vi "quiz3.vi"() -> ()   [LabVIEW 2020]
uses:
  <vilib>/Platform/TimedLoop/XDataNode/timing_clust.ctl
  <vilib>/Platform/TimedLoop/XDataNode/nitl_modes.ctl
  <vilib>/Platform/TimedLoop/XDataNode/wakeup.ctl
  enum.ctl
  <vilib>/Utility/file.llb/Read Delimited Spreadsheet (string).vi
  <vilib>/platform/TimedLoop/XDataNode/XDataNode.xnode
  <vilib>/Platform/TimedLoop/XDataNode/XDNodeRunTimeDep.lvlib
panel:
  out "Tab Control 2":enum32{"Login", "Registro", "Inicio"}(tab)
  in  "Enviar 2":bool
  in  "Usuario 2":string
  in  "Contraseña3":string
  out "Usuarios Eliminados 2":string[](array[string])
  out "Boolean 2":bool
  in  "Borrar Usuario 2":string
  in  "Usuario Nuevo 2":string
  in  "Clave de Usuario Nuevo 2":string
  in  "guardar 2":bool
  in  "Volver 2":bool
  in  "Borrar 2":bool
  in  "Volver a login 2":bool
  in  "Seleccione la secuencia":bool[][](array[boolean])
  out "Indicador por filas":bool[](array[boolean])
  out "Tab Control":enum32{"Login", "Registro", "Inicio"}(tab)
  in  "OK Button":bool
  in  "Usuario":string
  in  "Contraseña 2":string
  out "Boolean":bool
  in  "Borrar Usuario":string
  in  "Usuario Nuevo":string
  in  "Clave de Usuario Nuevo":string
  in  "guardar":bool
  in  "Volver":bool
  in  "Borrar":bool
  in  "Usuarios Eliminados":string[](array[string])
  in  "Volver a login":bool
  in  "Seleccione la secuencia":bool[][](array[boolean])
  out "Indicador por filas":bool[](array[boolean])
  # "Usuario"
  # "Contraseña"
  # "Usuarios Eliminados"
  # "Barrra de led interactiva"
  # "Contraseña"
  # "Barrra de led interactiva"
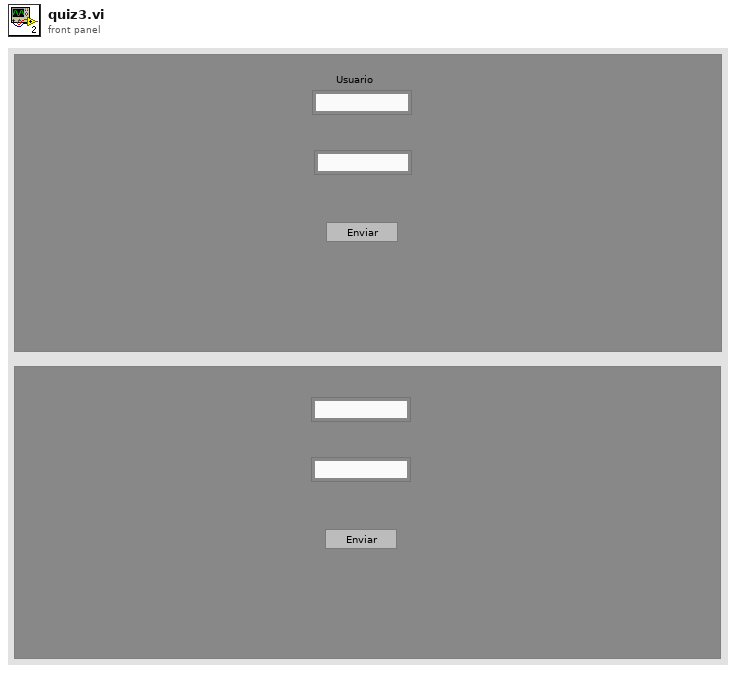
[diagram p1: front panel]
types:
  T1 = typedef "enum.ctl" = enum16{"login", "registro", "inicio"}
  T2 = enum16{"open", "replace", "create", "open or create", "replace or create", "replace or create with confirmation"}
  T3 = typedef "XDNodeRunTimeDep.lvlib/timing_clust.ctl" = cluster{"Expected End [f-1]":u64, "Actual End [f-1]":u64, "Finished Late? [f-1]":bool, "Expected End [i-1]":u64, "Actual End [i-1]":u64, "Finished Late? [i-1]":bool, "Expected Start [i]":u64, "Actual Start [i]":u64, "Expected Start [f]":u64, "Actual Start [f]":u64, "Source Name":string, "Structure Name":string, "Period":i64, "Deadline":i64, "Offset":i64, "Start":i64, "Priority":i32, "Timeout":i32, "Mode":T4, "Wakeup Reason":T5, "Error":errorcluster, "Source Type":string, "Secondary Source Type":string, "Global End Time":u64, "Global Start Time":u64, "Frame Duration":u64, "Iteration Duration":u64, "Assigned CPU":i32, "I/O Scan Engine Mode":u32}
  T4 = typedef "XDNodeRunTimeDep.lvlib/nitl_modes.ctl" = enum32{"No Change", "Process missed periods, maintain original phase", "Discard missed periods, maintain original phase", "Process missed periods, ignore original phase", "Discard missed periods, ignore original phase"}
  T5 = typedef "XDNodeRunTimeDep.lvlib/wakeup.ctl" = enum32{"Normal", "Aborted", "Asynchronous wakeup", "Timing source error", "Timed loop error", "Timeout"}
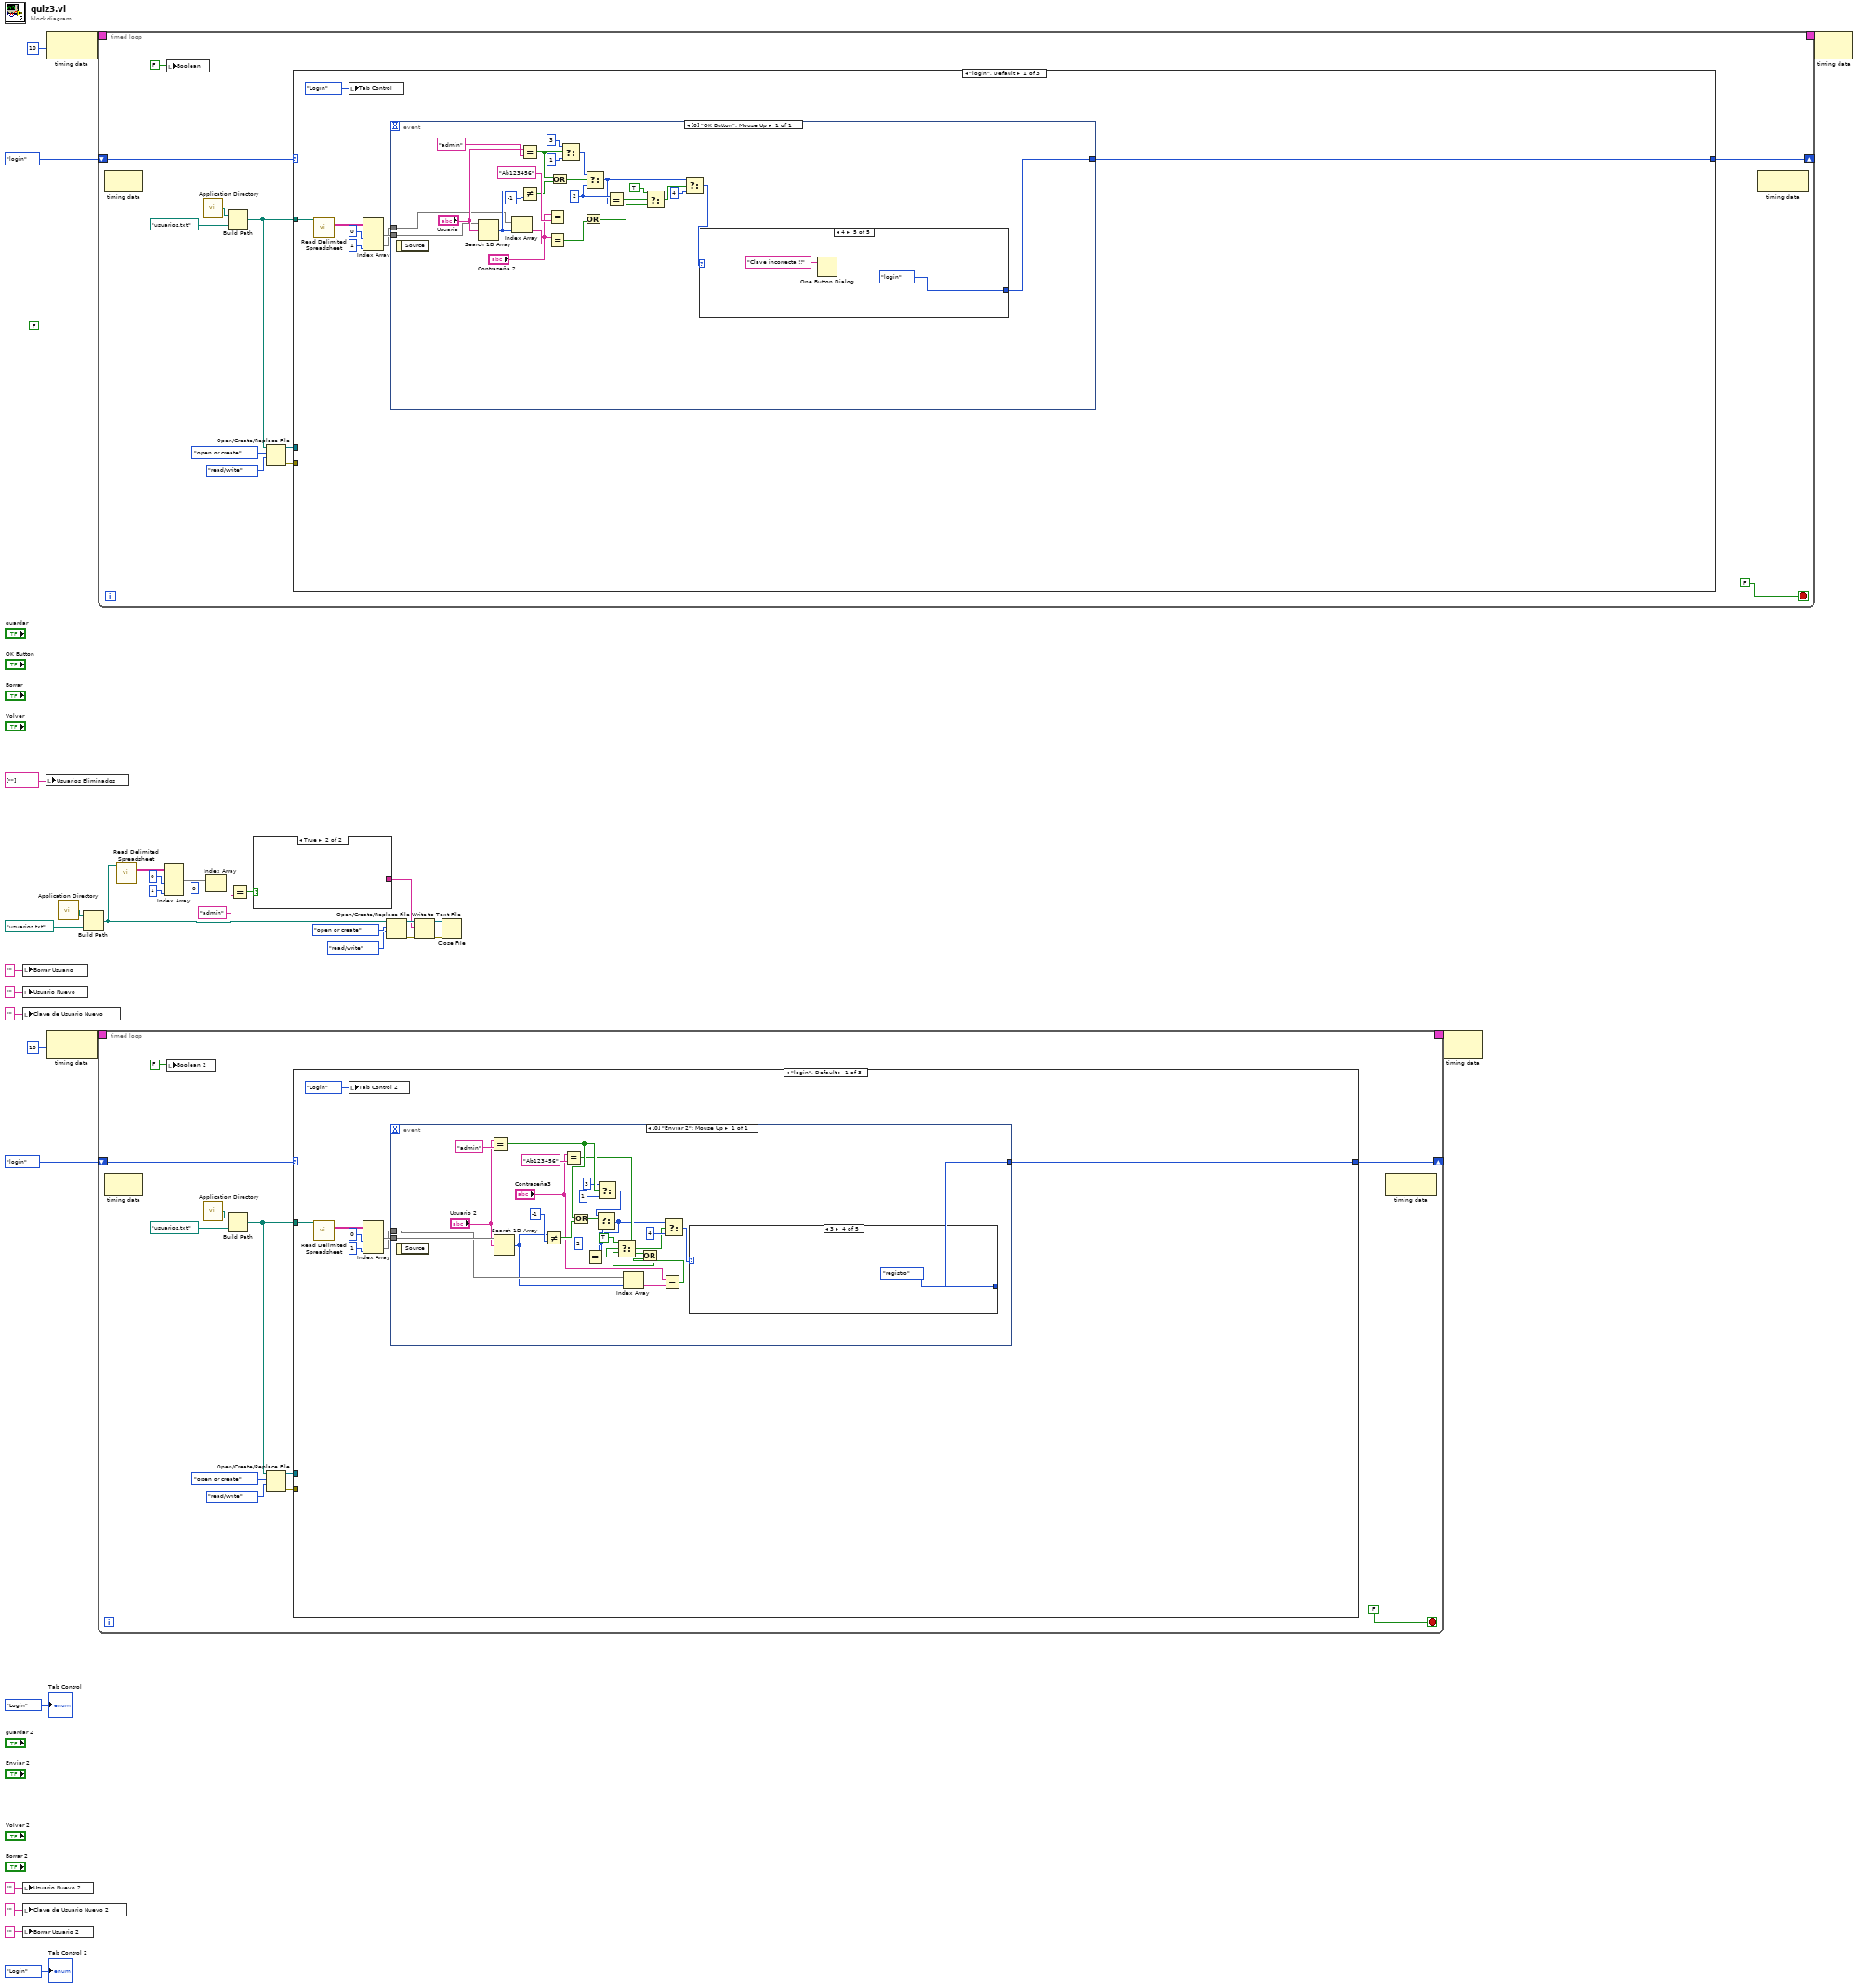
[diagram p0: block diagram]
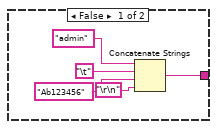
[diagram p2: hidden frame]
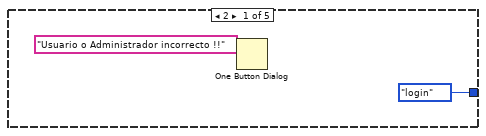
[diagram p3: hidden frame]
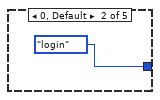
[diagram p4: hidden frame]
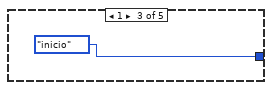
[diagram p5: hidden frame]
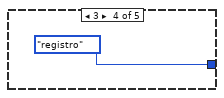
[diagram p6: hidden frame]
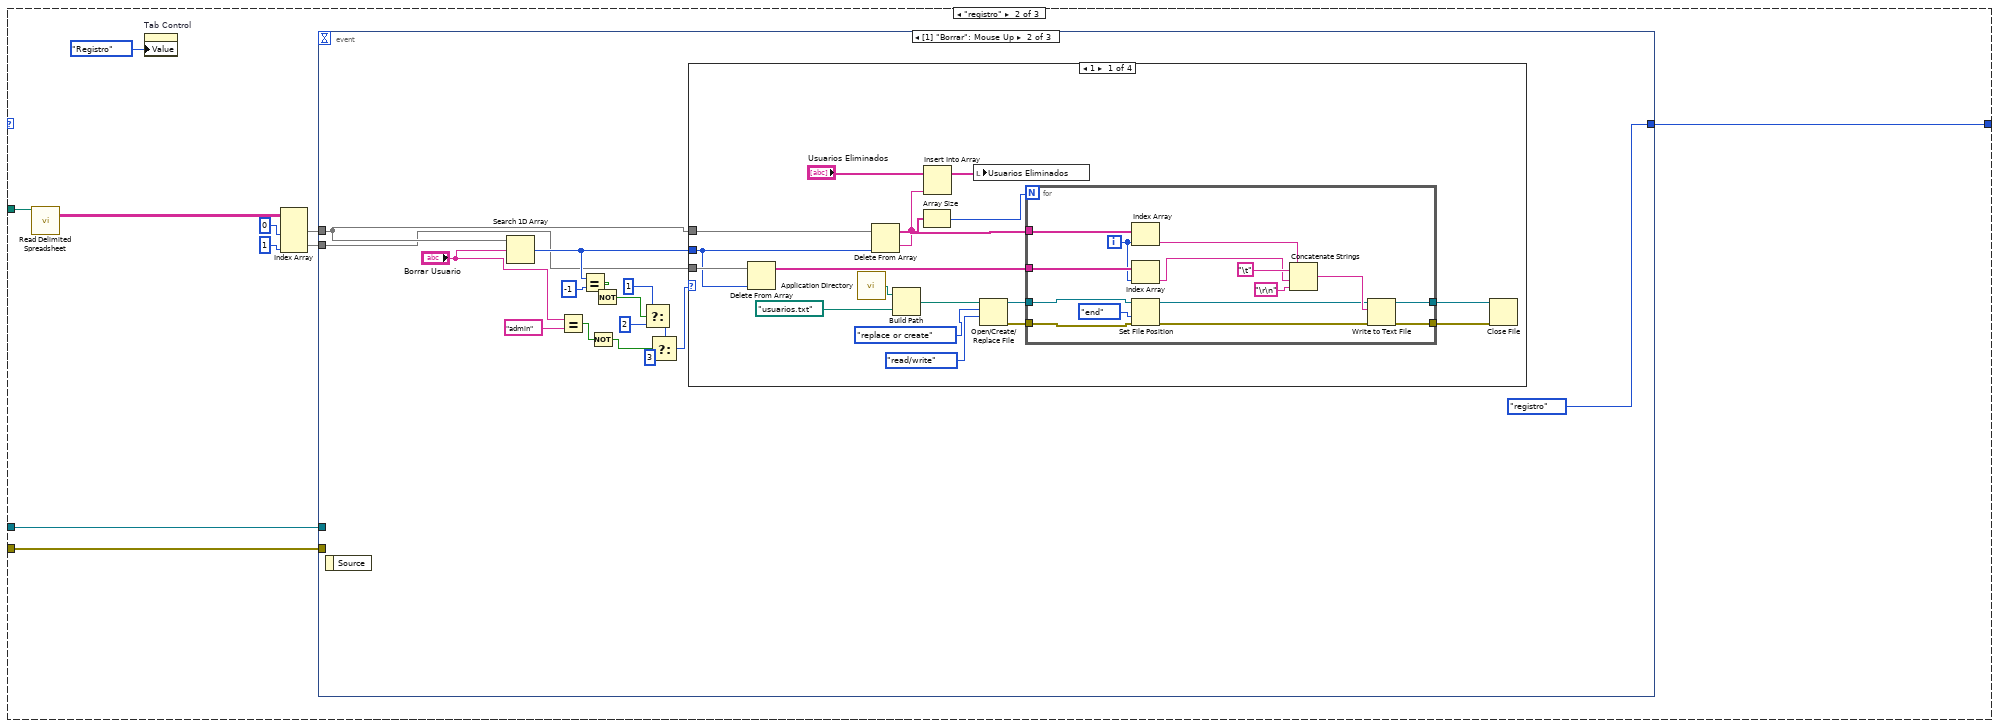
[diagram p7: hidden frame]
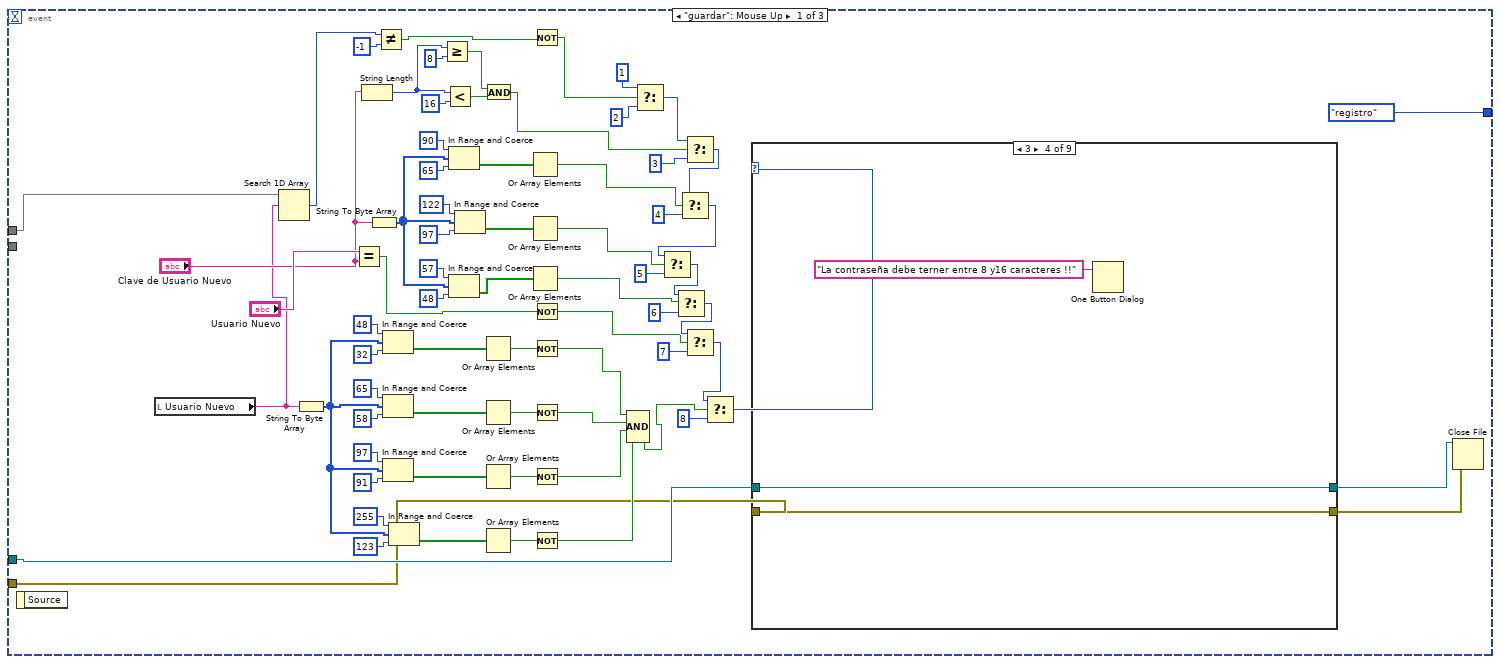
[diagram p8: hidden frame]
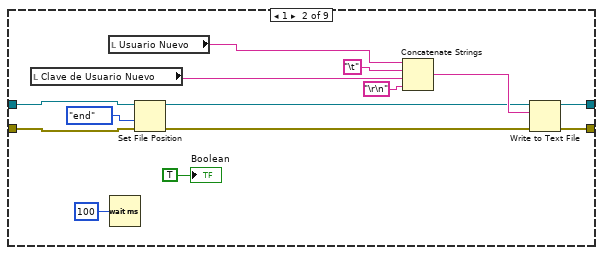
[diagram p10: hidden frame]
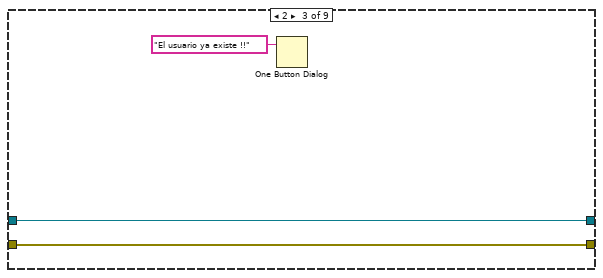
[diagram p11: hidden frame]
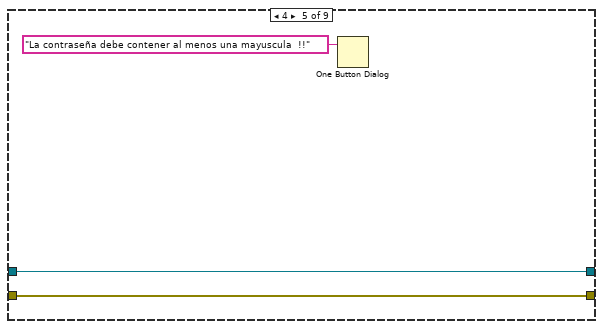
[diagram p12: hidden frame]
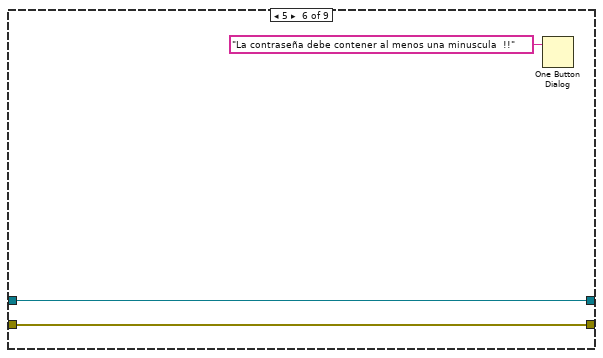
[diagram p13: hidden frame]
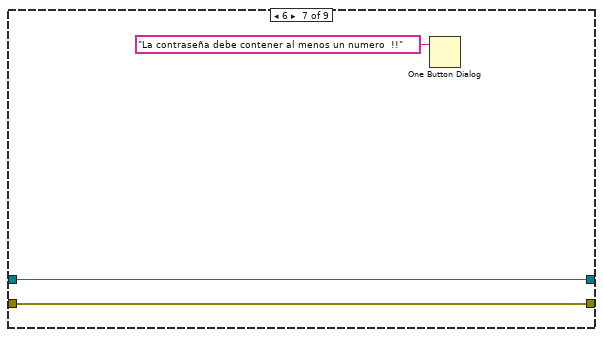
[diagram p14: hidden frame]
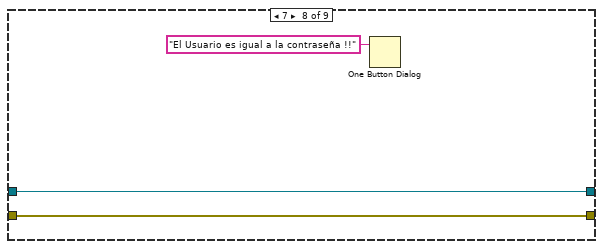
[diagram p15: hidden frame]
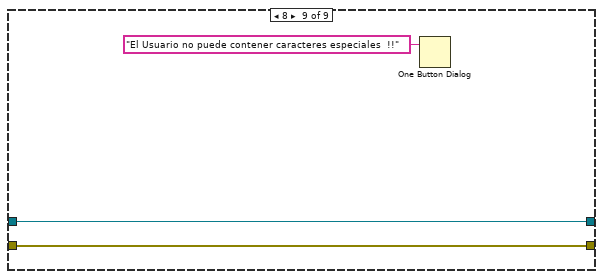
[diagram p16: hidden frame]
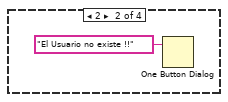
[diagram p17: hidden frame]
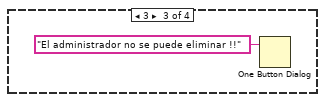
[diagram p18: hidden frame]
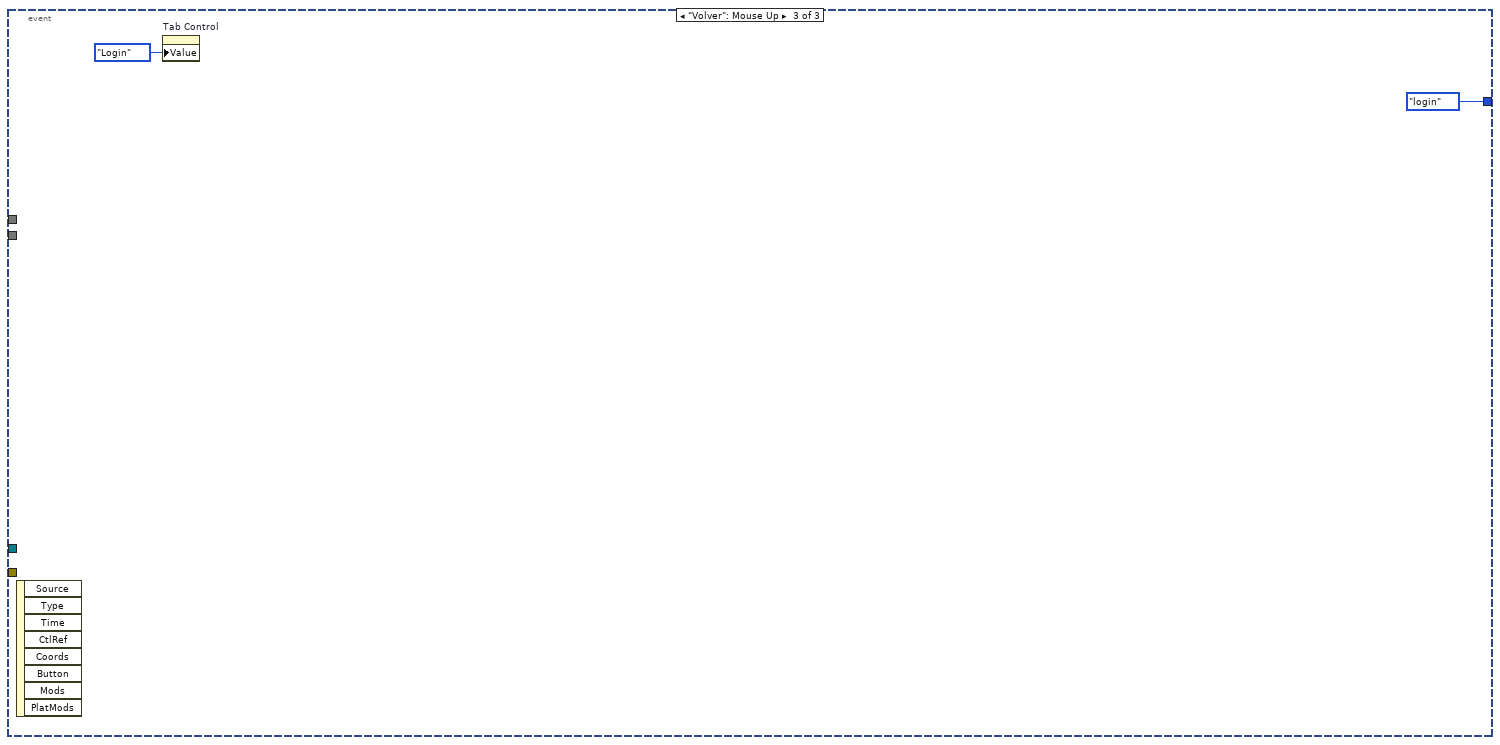
[diagram p20: hidden frame]
diagram:
  (unwired) FALSE ("Visible")
  n1 = local write "Borrar Usuario"("" ("Borrar Usuario")) -> ()
  n2 = local write "Usuario Nuevo"("" ("Usuario Nuevo")) -> ()
  n3 = local write "Clave de Usuario Nuevo"("" ("Clave de Usuario Nuevo")) -> ()
  n4 = local write "Usuario Nuevo 2"("" ("Usuario Nuevo 2")) -> ()
  n5 = local write "Clave de Usuario Nuevo 2"("" ("Clave de Usuario Nuevo 2")) -> ()
  n6 = local write "Borrar Usuario 2"("" ("Borrar Usuario 2")) -> ()
  n7 = local write "Usuarios Eliminados"(string[] [""] ("Usuarios Eliminados")) -> ()
  n8 = node-c288(i64 10 ("Period")) -> (w35:T3)
  n9 = node-c288(i64 10 ("Period")) -> (w9:T3)
  n10 = call <vilib>:"Application Directory.vi"() -> ("Application Directory"=w28:path)
  n11 = Build Path(base path=w28, name or relative path=path "usuarios.txt" ("file path (use dialog)")) -> (appended path=w19:path)
  n12 = timed-loop {
    timing: w35 -> [_]
    timing-out: [_] -> w34
    shift-right: [w44] -> _
    shift-left: enum."login" -> [w45]
    stop <- FALSE stop-if-true
    n13 = node-c288() -> ()  [unwired: 1 in, 1 out]
    n14 = local write "Boolean"(FALSE ("Boolean")) -> ()
    n15 = call <vilib>:"Application Directory.vi"() -> ("Application Directory"=w41:path)
    n16 = Build Path(base path=w41, name or relative path=path "usuarios.txt" ("file path (use dialog)")) -> (appended path=w37:path)
    n17 = Open/Create/Replace File(file path (use dialog)=w37, operation (0:open)=T2."open or create", access (0:read/write)=enum16{"read/write", "read-only", "write-only"}."read/write") -> (refnum out=w39:refnum<file>, error out=w38:errorcluster)  [unwired: 3 in, 1 out]
    n18 = case shown="\"login\", Default" w45 {
      tunnel: [w47 w94 w260] -> w44
      tunnel: w39 -> [_ w96 _]
      tunnel: w38 -> [_ w95 _]
      tunnel: w37 -> [w50 w90 _]
      frame "login", Default {
        n19 = call-poly <vilib>:"Read Delimited Spreadsheet.vi"("file path (dialog if empty)"=w50) -> ("all rows"=w53:string[][])  [unwired: 9 in, 5 out]
        n20 = local write "Tab Control"(enum32{"Login", "Registro", "Inicio"}."Login" ("Tab Control")) -> ()
        n21 = Index Array(array=w53, index (col) #1=0 ("disabled index (col)"), index (col) #2=1 ("index (col)")) -> (element #1=w49:string[], element #2=w48:string[])  [unwired: 2 in]
        n22 = event shown="[0] \"OK Button\": Mouse Up" {
          selector: _ -> [_]
          dyn-events: _ -> [_]
          timeout: _ -> [_]
          tunnel: w49 -> [w77]
          tunnel: w48 -> [w58]
          tunnel: [w55] -> w47
          event "OK Button": Mouse Up {
            w70 = 2 ("f")
            n23 = event-data() -> ()  [unwired: 1 in, 1 out]
            n24 = Search 1D Array(1D array=w77, element="Usuario") -> (index of element=w59:i32)  [unwired: 1 in]
            n25 = Index Array(array=w58, index=w59) -> (element=w57:string)
            n26 = Equal?(x="Usuario", y="admin") -> (x = y?=w62:bool)
            n27 = Not Equal?(x=w59, y=-1) -> (x != y?=w64:bool)
            n28 = Equal?(x="Contraseña 2", y="Ab123456") -> (x = y?=w56:bool)
            n29 = Equal?(x="Contraseña 2", y=w57) -> (x = y?=w72:bool)
            n30 = Or(x=w62, y=w64) -> (x .or. y?=w75:bool)
            n31 = Select(t=3 ("f"), s=w62, f=1) -> (s? t:f=w73:i32)
            n32 = Or(x=w56, y=w72) -> (x .or. y?=w66:bool)
            n33 = Select(t=w73, s=w75, f=w70) -> (s? t:f=w69:i32)
            n34 = Equal?(x=w70, y=w69) -> (x = y?=w68:bool)
            n35 = Select(t=TRUE, s=w68, f=w66) -> (s? t:f=w65:bool)
            n36 = Select(t=w69, s=w65, f=4) -> (s? t:f=w63:i32)
            n37 = case shown="4" w63 {
              tunnel: [enum."login" enum."login" enum."inicio" enum."registro" enum."login"] -> w55
              frame 2 {
                n38 = One Button Dialog(message="Usuario o Administrador incorrecto !!") -> ()  [unwired: 1 in, 1 out]
              }
              frame 0, Default {
              }
              frame 1 {
              }
              frame 3 {
              }
              frame 4 {
                n39 = One Button Dialog(message="Clave incorrecta !!") -> ()  [unwired: 1 in, 1 out]
              }
            }
          }
        }
      }
      frame "registro" {
        n40 = call-poly <vilib>:"Read Delimited Spreadsheet.vi"("file path (dialog if empty)"=w90) -> ("all rows"=w93:string[][])  [unwired: 9 in, 5 out]
        n41 = property on="Tab Control" class="TabCtl (strict)"("Value"=enum32{"Login", "Registro", "Inicio"}."Registro" ("Tab Control")) -> ()  [unwired: 2 in, 2 out]
        n42 = Index Array(array=w93, index (col) #1=0 ("disabled index (col)"), index (col) #2=1 ("index (col)")) -> (element #1=w89:string[], element #2=w88:string[])  [unwired: 2 in]
        n43 = event shown="[1] \"Borrar\": Mouse Up" {
          selector: _ -> [_ _ _]
          dyn-events: _ -> [_ _ _]
          timeout: _ -> [_ _ _]
          tunnel: w96 -> [w101 _ _]
          tunnel: w95 -> [w100 _ _]
          tunnel: [enum."registro" enum."registro" enum."login"] -> w94
          tunnel: w89 -> [w148 w220 _]
          tunnel: w88 -> [_ w218 _]
          event "guardar": Mouse Up {
            n44 = event-data() -> ()  [unwired: 1 in, 1 out]
            n45 = local read "Usuario Nuevo"() -> (w129:string)
            n46 = Search 1D Array(1D array=w148, element=w129) -> (index of element=w149:i32)  [unwired: 1 in]
            n47 = String To Byte Array(string=w129) -> (unsigned byte array=w128:u8[])
            n48 = Equal?(x="Usuario Nuevo", y="Clave de Usuario Nuevo") -> (x = y?=w154:bool)
            n49 = String Length(string="Clave de Usuario Nuevo") -> (length=w166:i32)
            n50 = String To Byte Array(string="Clave de Usuario Nuevo") -> (unsigned byte array=w136:u8[])
            n51 = Not Equal?(x=w149, y=-1) -> (x != y?=w147:bool)
            n52 = In Range and Coerce(upper limit=u8 48 ("lower limit"), x=w128, lower limit=u8 32) -> (In Range?=w144:bool[])  [unwired: 1 out]
            n53 = In Range and Coerce(upper limit=u8 65 ("lower limit"), x=w128, lower limit=u8 58) -> (In Range?=w135:bool[])  [unwired: 1 out]
            n54 = In Range and Coerce(upper limit=u8 97 ("lower limit"), x=w128, lower limit=u8 91) -> (In Range?=w134:bool[])  [unwired: 1 out]
            n55 = In Range and Coerce(upper limit=u8 255 ("lower limit"), x=w128, lower limit=u8 123) -> (In Range?=w133:bool[])  [unwired: 1 out]
            n56 = Greater Or Equal?(x=w166, y=8) -> (x >= y?=w167:bool)
            n57 = Less?(x=w166, y=16) -> (x < y?=w164:bool)
            n58 = In Range and Coerce(upper limit=u8 90, x=w136, lower limit=u8 65) -> (In Range?=w158:bool[])  [unwired: 1 out]
            n59 = In Range and Coerce(upper limit=u8 57, x=w136, lower limit=u8 48) -> (In Range?=w161:bool[])  [unwired: 1 out]
            n60 = In Range and Coerce(upper limit=u8 122, x=w136, lower limit=u8 97) -> (In Range?=w155:bool[])  [unwired: 1 out]
            n61 = Or Array Elements(Boolean array=w144) -> (logical OR=w143:bool)
            n62 = Or Array Elements(Boolean array=w135) -> (logical OR=w132:bool)
            n63 = Or Array Elements(Boolean array=w134) -> (logical OR=w131:bool)
            n64 = Or Array Elements(Boolean array=w133) -> (logical OR=w130:bool)
            n65 = And(x=w167, y=w164) -> (x .and. y?=w112:bool)
            n66 = Or Array Elements(Boolean array=w158) -> (logical OR=w111:bool)
            n67 = Or Array Elements(Boolean array=w155) -> (logical OR=w110:bool)
            n68 = Or Array Elements(Boolean array=w161) -> (logical OR=w109:bool)
            n69 = Not(x=w147) -> (.not. x?=w113:bool)
            n70 = Not(x=w154) -> (.not. x?=w108:bool)
            n71 = Not(x=w143) -> (.not. x?=w107:bool)
            n72 = Not(x=w132) -> (.not. x?=w106:bool)
            n73 = Not(x=w131) -> (.not. x?=w105:bool)
            n74 = Not(x=w130) -> (.not. x?=w104:bool)
            n75 = Compound Arithmetic op=AND(w107, w106, w105, w104) -> (w103:bool)
            n76 = Select(t=1 ("y"), s=w113, f=2) -> (s? t:f=w124:i32)
            n77 = Select(t=w124, s=w112, f=3) -> (s? t:f=w123:i32)
            n78 = Select(t=w123, s=w111, f=4) -> (s? t:f=w120:i32)
            n79 = Select(t=w120, s=w110, f=5) -> (s? t:f=w118:i32)
            n80 = Select(t=w118, s=w109, f=6) -> (s? t:f=w116:i32)
            n81 = Select(t=w116, s=w108, f=7) -> (s? t:f=w114:i32)
            n82 = Select(t=w114, s=w103, f=8) -> (s? t:f=w102:i32)
            n83 = case shown="3" w102 {
              tunnel: [w170 w178 w187 w189 w192 w195 w198 w201 w204] -> w99
              tunnel: [w169 w177 w186 w188 w191 w194 w197 w200 w203] -> w98
              tunnel: w101 -> [w170 w175 w187 w189 w192 w195 w198 w201 w204]
              tunnel: w100 -> [w169 w176 w186 w188 w191 w194 w197 w200 w203]
              frame 0, Default {
              }
              frame 1 {
                n84 = local read "Clave de Usuario Nuevo"() -> (w171:string)
                n85 = local read "Usuario Nuevo"() -> (w172:string)
                n86 = Wait (ms)(milliseconds to wait=u32 100) -> ()  [unwired: 1 out]
                n87 = Set File Position(refnum=w175, from (0:start)=enum16{"start", "end", "current"}."end", error in=w176) -> (refnum out=w181:refnum<file>, error out=w180:errorcluster)  [unwired: 1 in]
                n88 = Concatenate Strings(w172, "\t", w171, "\r\n") -> (w183:string)
                n89 = Write to Text File(file (use dialog)=w181, text=w183, error in=w180) -> (refnum out=w178:refnum<file>, error out=w177:errorcluster)  [unwired: 1 in, 1 out]
                "Boolean" <- TRUE ("Boolean")
              }
              frame 2 {
                n90 = One Button Dialog(message="El usuario ya existe !!") -> ()  [unwired: 1 in, 1 out]
              }
              frame 3 {
                n91 = One Button Dialog(message="La contraseña debe terner entre 8 y16 caracteres !!") -> ()  [unwired: 1 in, 1 out]
              }
              frame 4 {
                n92 = One Button Dialog(message="La contraseña debe contener al menos una mayuscula  !!") -> ()  [unwired: 1 in, 1 out]
              }
              frame 5 {
                n93 = One Button Dialog(message="La contraseña debe contener al menos una minuscula  !!") -> ()  [unwired: 1 in, 1 out]
              }
              frame 6 {
                n94 = One Button Dialog(message="La contraseña debe contener al menos un numero  !!") -> ()  [unwired: 1 in, 1 out]
              }
              frame 7 {
                n95 = One Button Dialog(message="El Usuario es igual a la contraseña !!") -> ()  [unwired: 1 in, 1 out]
              }
              frame 8 {
                n96 = One Button Dialog(message="El Usuario no puede contener caracteres especiales  !!") -> ()  [unwired: 1 in, 1 out]
              }
            }
            n97 = Close File(refnum=w99, error in=w98) -> ()  [unwired: 2 out]
          }
          event "Borrar": Mouse Up {
            n98 = event-data() -> ()  [unwired: 1 in, 1 out]
            n99 = Search 1D Array(1D array=w220, element="Borrar Usuario") -> (index of element=w219:i32)  [unwired: 1 in]
            n100 = Equal?(x="Borrar Usuario", y="admin") -> (x = y?=w207:bool)
            n101 = Equal?(x=w219, y=-1) -> (x = y?=w208:bool)
            n102 = Not(x=w207) -> (.not. x?=w211:bool)
            n103 = Not(x=w208) -> (.not. x?=w214:bool)
            n104 = Select(t=1 ("y"), s=w214, f=2) -> (s? t:f=w210:i32)
            n105 = Select(t=w210, s=w211, f=3) -> (s? t:f=w206:i32)
            n106 = case shown="1" w206 {
              tunnel: w220 -> [w239 _ _ _]
              tunnel: w219 -> [w237 _ _ _]
              tunnel: w218 -> [w238 _ _ _]
              frame 1 {
                n107 = Delete From Array(array=w238, index=w237) -> (array with subset deleted=w234:string[])  [unwired: 1 in, 1 out]
                n108 = call <vilib>:"Application Directory.vi"() -> ("Application Directory"=w231:path)
                n109 = Delete From Array(array=w239, index=w237) -> (deleted portion=w224:string, array with subset deleted=w235:string[])  [unwired: 1 in]
                n110 = Build Path(base path=w231, name or relative path=path "usuarios.txt" ("file path (use dialog)")) -> (appended path=w229:path)
                n111 = Array Size(array=w235) -> (size(s)=w236:i32)
                n112 = Insert Into Array(array="Usuarios Eliminados", new element=w224) -> (w222:string[])  [unwired: 1 in]
                n113 = local write "Usuarios Eliminados"(w222) -> ()
                n114 = Open/Create/Replace File(file path (use dialog)=w229, operation (0:open)=T2."replace or create", access (0:read/write)=enum16{"read/write", "read-only", "write-only"}."read/write") -> (refnum out=w226:refnum<file>, error out=w225:errorcluster)  [unwired: 3 in, 1 out]
                n115 = for {
                  N: w236 -> [_]
                  tunnel: w235 -> [w252]
                  tunnel: w234 -> [w250]
                  tunnel: [w244] -> w228
                  tunnel: [w243] -> w227
                  tunnel: w226 -> [w242]
                  tunnel: w225 -> [w241]
                  i -> [w249]
                  n116 = Index Array "Index Array"(array=w252, index=w249) -> (element=w251:string)
                  n117 = Index Array(array=w250, index=w249) -> (element=w248:string)
                  n118 = Set File Position(refnum=w242, from (0:start)=enum16{"start", "end", "current"}."end", error in=w241) -> (refnum out=w246:refnum<file>, error out=w245:errorcluster)  [unwired: 1 in]
                  n119 = Concatenate Strings(w251, "\t", w248, "\r\n") -> (w247:string)
                  n120 = Write to Text File(file (use dialog)=w246, text=w247, error in=w245) -> (refnum out=w244:refnum<file>, error out=w243:errorcluster)  [unwired: 1 in, 1 out]
                }
                n121 = Close File(refnum=w228, error in=w227) -> ()  [unwired: 2 out]
              }
              frame 2 {
                n122 = One Button Dialog(message="El Usuario no existe !!") -> ()  [unwired: 1 in, 1 out]
              }
              frame 3 {
                n123 = One Button Dialog(message="El administrador no se puede eliminar !!") -> ()  [unwired: 1 in, 1 out]
              }
              frame 0, Default {
              }
            }
          }
          event "Volver": Mouse Up {
            n124 = event-data() -> ()  [unwired: 1 in, 8 out]
            n125 = property on="Tab Control" class="TabCtl (strict)"("Value"=enum32{"Login", "Registro", "Inicio"}."Login" ("Tab Control")) -> ()  [unwired: 2 in, 2 out]
          }
        }
      }
      frame "inicio" {
        n126 = local write "Tab Control"(enum32{"Login", "Registro", "Inicio"}."Inicio" ("Tab Control")) -> ()
        n127 = while {
          shift-right: [w264] -> _
          shift-left: 0 -> [w269]
          stop <- "Volver a login" stop-if-true
          n128 = Increment(x=w269) -> (x+1=w267:i32)
          n129 = Wait (ms)(milliseconds to wait=u32 150) -> ()  [unwired: 1 out]
          n130 = Less Or Equal?(x=w267, y=9) -> (x <= y?=w268:bool)
          n131 = Select(t=w267, s=w268, f=0) -> (s? t:f=w264:i32)
          n132 = Index Array(array="Seleccione la secuencia", index (row)=w264) -> (element=→"Indicador por filas":bool[])  [unwired: 1 in]
        }
        n133 = event shown="[0] \"Volver a login\": Mouse Up" {
          selector: _ -> [_]
          dyn-events: _ -> [_]
          timeout: _ -> [_]
          tunnel: [enum."login"] -> w260
          event "Volver a login": Mouse Up {
            n134 = event-data() -> ()  [unwired: 1 in, 8 out]
            n135 = local write "Tab Control"(enum32{"Login", "Registro", "Inicio"}."Login" ("Tab Control")) -> ()
          }
        }
      }
    }
    n136 = node-c288() -> ()  [unwired: 1 in, 1 out]
  }
  n137 = timed-loop {
    timing: w9 -> [_]
    timing-out: [_] -> w8
    shift-right: [w284] -> _
    shift-left: enum."login" -> [w285]
    stop <- FALSE stop-if-true
    n138 = node-c288() -> ()  [unwired: 1 in, 1 out]
    n139 = local write "Boolean 2"(FALSE ("Boolean")) -> ()
    n140 = call <vilib>:"Application Directory.vi"() -> ("Application Directory"=w281:path)
    n141 = Build Path(base path=w281, name or relative path=path "usuarios.txt" ("file path (use dialog)")) -> (appended path=w277:path)
    n142 = Open/Create/Replace File(file path (use dialog)=w277, operation (0:open)=T2."open or create", access (0:read/write)=enum16{"read/write", "read-only", "write-only"}."read/write") -> (refnum out=w279:refnum<file>, error out=w278:errorcluster)  [unwired: 3 in, 1 out]
    n143 = case shown="\"login\", Default" w285 {
      tunnel: [w287 w334 w501] -> w284
      tunnel: w279 -> [_ w336 _]
      tunnel: w278 -> [_ w335 _]
      tunnel: w277 -> [w290 w330 _]
      frame "login", Default {
        n144 = call-poly <vilib>:"Read Delimited Spreadsheet.vi"("file path (dialog if empty)"=w290) -> ("all rows"=w293:string[][])  [unwired: 9 in, 5 out]
        n145 = local write "Tab Control 2"(enum32{"Login", "Registro", "Inicio"}."Login" ("Tab Control")) -> ()
        n146 = Index Array(array=w293, index (col) #1=0 ("disabled index (col)"), index (col) #2=1 ("index (col)")) -> (element #1=w289:string[], element #2=w288:string[])  [unwired: 2 in]
        n147 = event shown="[0] \"Enviar 2\": Mouse Up" {
          selector: _ -> [_]
          dyn-events: _ -> [_]
          timeout: _ -> [_]
          tunnel: w289 -> [w318]
          tunnel: w288 -> [w308]
          tunnel: [w315] -> w287
          event "Enviar 2": Mouse Up {
            w300 = 2 ("f")
            n148 = event-data() -> ()  [unwired: 1 in, 1 out]
            n149 = Equal?(x="Usuario 2", y="admin") -> (x = y?=w312:bool)
            n150 = Search 1D Array(1D array=w318, element="Usuario 2") -> (index of element=w305:i32)  [unwired: 1 in]
            n151 = Not Equal?(x=w305, y=-1) -> (x != y?=w314:bool)
            n152 = Equal?(x="Contraseña3", y="Ab123456") -> (x = y?=w303:bool)
            n153 = Or(x=w312, y=w314) -> (x .or. y?=w313:bool)
            n154 = Select(t=3 ("f"), s=w312, f=1) -> (s? t:f=w309:i32)
            n155 = Select(t=w309, s=w313, f=w300) -> (s? t:f=w299:i32)
            n156 = Equal?(x=w300, y=w299) -> (x = y?=w298:bool)
            n157 = Index Array(array=w308, index=w305) -> (element=w306:string)
            n158 = Equal?(x="Contraseña3", y=w306) -> (x = y?=w304:bool)
            n159 = Or(x=w303, y=w304) -> (x .or. y?=w296:bool)
            n160 = Select(t=TRUE, s=w298, f=w296) -> (s? t:f=w295:bool)
            n161 = Select(t=w299, s=w295, f=4) -> (s? t:f=w301:i32)
            n162 = case shown="3" w301 {
              tunnel: [enum."login" enum."login" enum."inicio" enum."registro" enum."login"] -> w315
              frame 2 {
                n163 = One Button Dialog(message="Usuario o Administrador incorrecto !!") -> ()  [unwired: 1 in, 1 out]
              }
              frame 0, Default {
              }
              frame 1 {
              }
              frame 3 {
              }
              frame 4 {
                n164 = One Button Dialog(message="Clave incorrecta !!") -> ()  [unwired: 1 in, 1 out]
              }
            }
          }
        }
      }
      frame "registro" {
        n165 = call-poly <vilib>:"Read Delimited Spreadsheet.vi"("file path (dialog if empty)"=w330) -> ("all rows"=w333:string[][])  [unwired: 9 in, 5 out]
        n166 = Index Array(array=w333, index (col) #1=0 ("disabled index (col)"), index (col) #2=1 ("index (col)")) -> (element #1=w329:string[], element #2=w328:string[])  [unwired: 2 in]
        n167 = property on="Tab Control 2" class="TabCtl (strict)"("Value"=enum32{"Login", "Registro", "Inicio"}."Registro" ("Tab Control")) -> ()  [unwired: 2 in, 2 out]
        n168 = event shown="[1] \"Borrar 2\": Mouse Up" {
          selector: _ -> [_ _ _]
          dyn-events: _ -> [_ _ _]
          timeout: _ -> [_ _ _]
          tunnel: w336 -> [w393 _ _]
          tunnel: w335 -> [w392 _ _]
          tunnel: [enum."registro" enum."registro" enum."login"] -> w334
          tunnel: w329 -> [w384 w460 _]
          tunnel: w328 -> [_ w458 _]
          event "guardar 2": Mouse Up {
            # "Usuario = contraseña"
            # "Numeros"
            # "minusculas"
            # "Usuarios iguales"
            # "Entre 8 y 16"
            # "mayusculas"
            n169 = event-data() -> ()  [unwired: 1 in, 1 out]
            n170 = local read "Usuario Nuevo 2"() -> (w365:string)
            n171 = Search 1D Array(1D array=w384, element=w365) -> (index of element=w385:i32)  [unwired: 1 in]
            n172 = String To Byte Array(string=w365) -> (unsigned byte array=w364:u8[])
            n173 = Equal?(x="Usuario Nuevo 2", y="Clave de Usuario Nuevo 2") -> (x = y?=w394:bool)
            n174 = String Length(string="Clave de Usuario Nuevo 2") -> (length=w406:i32)
            n175 = String To Byte Array(string="Clave de Usuario Nuevo 2") -> (unsigned byte array=w372:u8[])
            n176 = Not Equal?(x=w385, y=-1) -> (x != y?=w383:bool)
            n177 = In Range and Coerce(upper limit=u8 48 ("lower limit"), x=w364, lower limit=u8 32) -> (In Range?=w380:bool[])  [unwired: 1 out]
            n178 = In Range and Coerce(upper limit=u8 65 ("lower limit"), x=w364, lower limit=u8 58) -> (In Range?=w371:bool[])  [unwired: 1 out]
            n179 = In Range and Coerce(upper limit=u8 97 ("lower limit"), x=w364, lower limit=u8 91) -> (In Range?=w370:bool[])  [unwired: 1 out]
            n180 = In Range and Coerce(upper limit=u8 255 ("lower limit"), x=w364, lower limit=u8 123) -> (In Range?=w369:bool[])  [unwired: 1 out]
            n181 = Greater Or Equal?(x=w406, y=8) -> (x >= y?=w407:bool)
            n182 = Less?(x=w406, y=16) -> (x < y?=w404:bool)
            n183 = In Range and Coerce(upper limit=u8 90, x=w372, lower limit=u8 65) -> (In Range?=w398:bool[])  [unwired: 1 out]
            n184 = In Range and Coerce(upper limit=u8 57, x=w372, lower limit=u8 48) -> (In Range?=w401:bool[])  [unwired: 1 out]
            n185 = In Range and Coerce(upper limit=u8 122, x=w372, lower limit=u8 97) -> (In Range?=w395:bool[])  [unwired: 1 out]
            n186 = Or Array Elements(Boolean array=w380) -> (logical OR=w379:bool)
            n187 = Or Array Elements(Boolean array=w371) -> (logical OR=w368:bool)
            n188 = Or Array Elements(Boolean array=w370) -> (logical OR=w367:bool)
            n189 = Or Array Elements(Boolean array=w369) -> (logical OR=w366:bool)
            n190 = And(x=w407, y=w404) -> (x .and. y?=w359:bool)
            n191 = Or Array Elements(Boolean array=w398) -> (logical OR=w357:bool)
            n192 = Or Array Elements(Boolean array=w395) -> (logical OR=w352:bool)
            n193 = Or Array Elements(Boolean array=w401) -> (logical OR=w350:bool)
            n194 = Not(x=w383) -> (.not. x?=w363:bool)
            n195 = Not(x=w394) -> (.not. x?=w347:bool)
            n196 = Not(x=w379) -> (.not. x?=w345:bool)
            n197 = Not(x=w368) -> (.not. x?=w344:bool)
            n198 = Not(x=w367) -> (.not. x?=w343:bool)
            n199 = Not(x=w366) -> (.not. x?=w342:bool)
            n200 = Compound Arithmetic op=AND(w345, w344, w343, w342) -> (w340:bool)
            n201 = Select(t=1 ("y"), s=w363, f=2) -> (s? t:f=w358:i32)
            n202 = Select(t=w358, s=w359, f=3) -> (s? t:f=w356:i32)
            n203 = Select(t=w356, s=w357, f=4) -> (s? t:f=w353:i32)
            n204 = Select(t=w353, s=w352, f=5) -> (s? t:f=w349:i32)
            n205 = Select(t=w349, s=w350, f=6) -> (s? t:f=w346:i32)
            n206 = Select(t=w346, s=w347, f=7) -> (s? t:f=w339:i32)
            n207 = Select(t=w339, s=w340, f=8) -> (s? t:f=w338:i32)
            n208 = case shown="1" w338 {
              tunnel: [w410 w418 w427 w429 w432 w435 w438 w441 w444] -> w390
              tunnel: [w409 w417 w426 w428 w431 w434 w437 w440 w443] -> w389
              tunnel: w393 -> [w410 w414 w427 w429 w432 w435 w438 w441 w444]
              tunnel: w392 -> [w409 w415 w426 w428 w431 w434 w437 w440 w443]
              frame 0, Default {
              }
              frame 1 {
                n209 = Wait (ms)(milliseconds to wait=u32 100) -> ()  [unwired: 1 out]
                n210 = local read "Clave de Usuario Nuevo 2"() -> (w416:string)
                n211 = Set File Position(refnum=w414, from (0:start)=enum16{"start", "end", "current"}."end", error in=w415) -> (refnum out=w421:refnum<file>, error out=w420:errorcluster)  [unwired: 1 in]
                n212 = local read "Usuario Nuevo 2"() -> (w413:string)
                n213 = Concatenate Strings(w413, "\t", w416, "\r\n") -> (w423:string)
                n214 = Write to Text File(file (use dialog)=w421, text=w423, error in=w420) -> (refnum out=w418:refnum<file>, error out=w417:errorcluster)  [unwired: 1 in, 1 out]
                "Boolean 2" <- TRUE ("Boolean")
              }
              frame 2 {
                n215 = One Button Dialog(message="El usuario ya existe !!") -> ()  [unwired: 1 in, 1 out]
              }
              frame 3 {
                n216 = One Button Dialog(message="La contraseña debe terner entre 8 y16 caracteres !!") -> ()  [unwired: 1 in, 1 out]
              }
              frame 4 {
                n217 = One Button Dialog(message="La contraseña debe contener al menos una mayuscula  !!") -> ()  [unwired: 1 in, 1 out]
              }
              frame 5 {
                n218 = One Button Dialog(message="La contraseña debe contener al menos una minuscula  !!") -> ()  [unwired: 1 in, 1 out]
              }
              frame 6 {
                n219 = One Button Dialog(message="La contraseña debe contener al menos un numero  !!") -> ()  [unwired: 1 in, 1 out]
              }
              frame 7 {
                n220 = One Button Dialog(message="El Usuario es igual a la contraseña !!") -> ()  [unwired: 1 in, 1 out]
              }
              frame 8 {
                n221 = One Button Dialog(message="El Usuario no puede contener caracteres especiales  !!") -> ()  [unwired: 1 in, 1 out]
              }
            }
            n222 = Close File(refnum=w390, error in=w389) -> ()  [unwired: 2 out]
          }
          event "Borrar 2": Mouse Up {
            n223 = event-data() -> ()  [unwired: 1 in, 1 out]
            n224 = Search 1D Array(1D array=w460, element="Borrar Usuario 2") -> (index of element=w459:i32)  [unwired: 1 in]
            n225 = Equal?(x="Borrar Usuario 2", y="admin") -> (x = y?=w450:bool)
            n226 = Equal?(x=w459, y=-1) -> (x = y?=w454:bool)
            n227 = Not(x=w450) -> (.not. x?=w449:bool)
            n228 = Not(x=w454) -> (.not. x?=w453:bool)
            n229 = Select(t=1 ("y"), s=w453, f=2) -> (s? t:f=w448:i32)
            n230 = Select(t=w448, s=w449, f=3) -> (s? t:f=w446:i32)
            n231 = case shown="1" w446 {
              tunnel: w460 -> [w480 _ _ _]
              tunnel: w459 -> [w478 _ _ _]
              tunnel: w458 -> [w479 _ _ _]
              frame 1 {
                n232 = Delete From Array(array=w479, index=w478) -> (array with subset deleted=w475:string[])  [unwired: 1 in, 1 out]
                n233 = local read "Usuarios Eliminados"() -> (w463:string[])
                n234 = call <vilib>:"Application Directory.vi"() -> ("Application Directory"=w472:path)
                n235 = Delete From Array(array=w480, index=w478) -> (deleted portion=w465:string, array with subset deleted=w476:string[])  [unwired: 1 in]
                n236 = Build Path(base path=w472, name or relative path=path "usuarios.txt" ("file path (use dialog)")) -> (appended path=w470:path)
                n237 = Array Size(array=w476) -> (size(s)=w477:i32)
                n238 = Insert Into Array(array=w463, new element=w465) -> (w464:string[])  [unwired: 1 in]
                n239 = local write "Usuarios Eliminados"(w464) -> ()
                n240 = Open/Create/Replace File(file path (use dialog)=w470, operation (0:open)=T2."replace or create", access (0:read/write)=enum16{"read/write", "read-only", "write-only"}."read/write") -> (refnum out=w467:refnum<file>, error out=w466:errorcluster)  [unwired: 3 in, 1 out]
                n241 = for {
                  N: w477 -> [_]
                  tunnel: w476 -> [w493]
                  tunnel: w475 -> [w491]
                  tunnel: [w485] -> w469
                  tunnel: [w484] -> w468
                  tunnel: w467 -> [w483]
                  tunnel: w466 -> [w482]
                  i -> [w490]
                  n242 = Index Array(array=w493, index=w490) -> (element=w492:string)
                  n243 = Index Array(array=w491, index=w490) -> (element=w489:string)
                  n244 = Set File Position(refnum=w483, from (0:start)=enum16{"start", "end", "current"}."end", error in=w482) -> (refnum out=w487:refnum<file>, error out=w486:errorcluster)  [unwired: 1 in]
                  n245 = Concatenate Strings(w492, "\t", w489, "\r\n") -> (w488:string)
                  n246 = Write to Text File(file (use dialog)=w487, text=w488, error in=w486) -> (refnum out=w485:refnum<file>, error out=w484:errorcluster)  [unwired: 1 in, 1 out]
                }
                n247 = local read "Usuarios Eliminados"() -> (→"Usuarios Eliminados 2":string[])
                n248 = Close File(refnum=w469, error in=w468) -> ()  [unwired: 2 out]
              }
              frame 2 {
                n249 = One Button Dialog(message="El Usuario no existe !!") -> ()  [unwired: 1 in, 1 out]
              }
              frame 3 {
                n250 = One Button Dialog(message="El administrador no se puede eliminar !!") -> ()  [unwired: 1 in, 1 out]
              }
              frame 0, Default {
              }
            }
          }
          event "Volver 2": Mouse Up {
            n251 = event-data() -> ()  [unwired: 1 in, 8 out]
            n252 = property on="Tab Control 2" class="TabCtl (strict)"("Value"=enum32{"Login", "Registro", "Inicio"}."Login" ("Tab Control")) -> ()  [unwired: 2 in, 2 out]
          }
        }
      }
      frame "inicio" {
        n253 = local write "Tab Control 2"(enum32{"Login", "Registro", "Inicio"}."Inicio" ("Tab Control")) -> ()
        n254 = while {
          shift-right: [w505] -> _
          shift-left: 0 -> [w510]
          stop <- "Volver a login 2" stop-if-true
          n255 = Increment(x=w510) -> (x+1=w508:i32)
          n256 = Wait (ms)(milliseconds to wait=u32 150) -> ()  [unwired: 1 out]
          n257 = Less Or Equal?(x=w508, y=9) -> (x <= y?=w509:bool)
          n258 = Select(t=w508, s=w509, f=0) -> (s? t:f=w505:i32)
          n259 = Index Array(array="Seleccione la secuencia", index (row)=w505) -> (element=→"Indicador por filas":bool[])  [unwired: 1 in]
        }
        n260 = event shown="[0] \"Volver a login 2\": Mouse Up" {
          selector: _ -> [_]
          dyn-events: _ -> [_]
          timeout: _ -> [_]
          tunnel: [enum."login"] -> w501
          event "Volver a login 2": Mouse Up {
            n261 = event-data() -> ()  [unwired: 1 in, 8 out]
            n262 = local write "Tab Control 2"(enum32{"Login", "Registro", "Inicio"}."Login" ("Tab Control")) -> ()
          }
        }
      }
    }
    n263 = node-c288() -> ()  [unwired: 1 in, 1 out]
  }
  n264 = call-poly <vilib>:"Read Delimited Spreadsheet.vi"("file path (dialog if empty)"=w19) -> ("all rows"=w22:string[][])  [unwired: 9 in, 5 out]
  n265 = Index Array(array=w22, index (col) #1=0 ("disabled index (col)"), index (col) #2=1 ("index (col)")) -> (element #1=w18:string[])  [unwired: 2 in, 1 out]
  n266 = Index Array(array=w18, index=0) -> (element=w16:string)
  n267 = Equal?(x=w16, y="admin" ("string")) -> (x = y?=w14:bool)
  n268 = case shown="True" w14 {
    tunnel: [w517 _] -> w13
    frame False {
      n269 = Concatenate Strings("admin" ("string"), "\t", "Ab123456" ("string"), "\r\n") -> (w517:string)
    }
    frame True {
    }
  }
  n270 = Open/Create/Replace File(file path (use dialog)=w19, operation (0:open)=T2."open or create", access (0:read/write)=enum16{"read/write", "read-only", "write-only"}."read/write") -> (refnum out=w26:refnum<file>, error out=w25:errorcluster)  [unwired: 3 in, 1 out]
  n271 = Write to Text File(file (use dialog)=w26, text=w13, error in=w25) -> (refnum out=w24:refnum<file>, error out=w23:errorcluster)  [unwired: 1 in, 1 out]
  n272 = Close File(refnum=w24, error in=w23) -> ()  [unwired: 2 out]
  n273 = node-c288(w8) -> ()  [unwired: 1 out]
  n274 = node-c288(w34) -> ()  [unwired: 1 out]
  "Tab Control" <- enum32{"Login", "Registro", "Inicio"}."Login" ("Tab Control")
  "Tab Control 2" <- enum32{"Login", "Registro", "Inicio"}."Login" ("Tab Control 2")
